vi "TestSetInWavePair.vi"(8 "error in (no error)":errorcluster) -> (0 "error out":errorcluster)   [LabVIEW 2019]
uses:
  <vilib>/addons/_JKI Toolkits/Caraya/classes/Test/Test.lvclass
  <vilib>/addons/_JKI Toolkits/Caraya/classes/Assert/Assert.lvclass
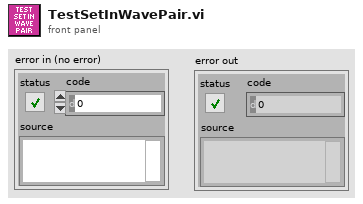
[diagram p1: front panel]
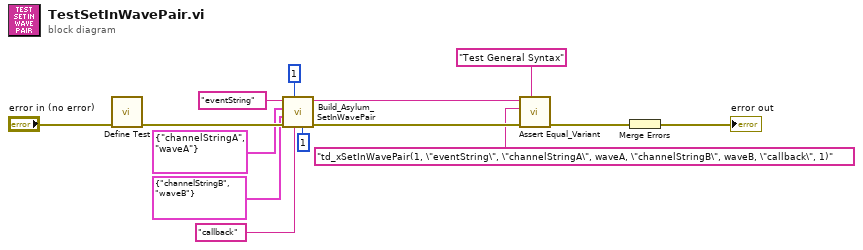
[diagram p0: block diagram]
diagram:
  n1 = call <vilib>:"Define Test.vi"("error in (no error)"="error in (no error)") -> ("error out"=w10:errorcluster)  [unwired: 10 in]
  n2 = call "Build_Asylum_SetInWavePair.vi"("decimation"=1, "callback"="callback", "whichBank"=1, "error in (no error)"=w10, "WaveB"=cluster{"channelString":string, "wave":string} {"channelString"="channelStringB", "wave"="waveB"} ("Wave"), "WaveA"=cluster{"channelString":string, "wave":string} {"channelString"="channelStringA", "wave"="waveA"} ("Wave"), "eventString"="eventString") -> ("error out"=w9:errorcluster, "Command"=w8:string)  [unwired: 3 in]
  n3 = call <vilib>:"Assert Equal_Variant.vi"("Label"="Test General Syntax", "error in (no error)"=w9, "Y"="td_xSetInWavePair(1, \"eventString\", \"channelStringA\", waveA, \"channelStringB\", waveB, \"callback\", 1)", "X"=w8) -> ("error out"=w12:errorcluster)  [unwired: 7 in]
  n4 = Merge Errors(w12) -> (→"error out":errorcluster)
